vi "Create CSVs.vi"(8 "error in (no error)":errorcluster, 10 "CSV config section":string="RAW", 11 "CSV File Name":string=" GPS RAW DATA.csv") -> (0 "error out":errorcluster, 3 "CSV refnum":path)   [LabVIEW 2025]
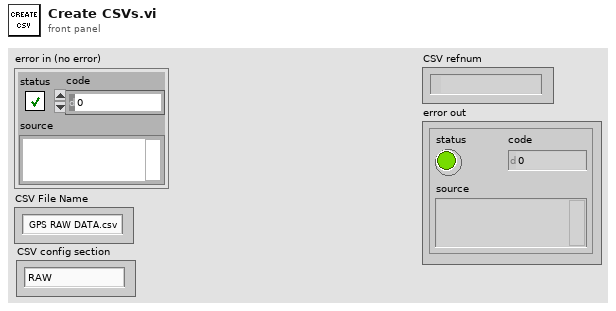
[diagram p1: front panel]
types:
  T1 = enum16{"open", "replace", "create", "open or create", "replace or create", "replace or create with confirmation"}
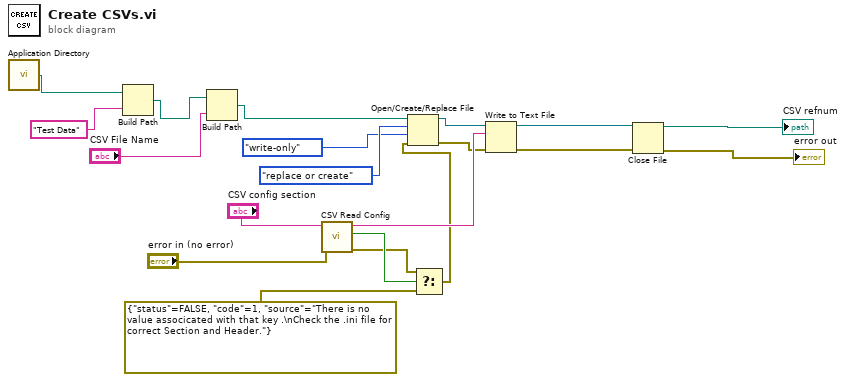
[diagram p0: block diagram]
diagram:
  n1 = call <vilib>:"Application Directory.vi"() -> ("Application Directory"=w20:path)
  n2 = Build Path(base path=w20, name or relative path="Test Data" ("regular expression")) -> (appended path=w15:path)
  n3 = Build Path(base path=w15, name or relative path="CSV File Name") -> (appended path=w14:path)
  n4 = call "CSV Read Config.vi"("error in (no error)"="error in (no error)", "CSV Section Name"="CSV config section") -> ("error out"=w1:errorcluster, "found?"=w4:bool, "Header"=w11:string)  [unwired: 7 in]
  n5 = Select(t=w1, s=w4, f=errorcluster {"status"=FALSE, "code"=1, "source"="There is no value associcated with that key .\nCheck the .ini file for correct Section and Header."} ("error out")) -> (s? t:f=w2:errorcluster)
  n6 = Open/Create/Replace File(file path (use dialog)=w14, error in=w2, operation (0:open)=T1."replace or create", access (0:read/write)=enum16{"read/write", "read-only", "write-only"}."write-only") -> (refnum out=w17:refnum<file>, error out=w7:errorcluster)  [unwired: 2 in, 1 out]
  n7 = Write to Text File(file (use dialog)=w17, text=w11, error in=w7) -> (refnum out=w10:refnum<file>, error out=w6:errorcluster)  [unwired: 1 in, 1 out]
  n8 = Close File(refnum=w10, error in=w6) -> (path=→"CSV refnum":path, error out=→"error out":errorcluster)
